vi "RGA queue listener (SubVI).vi"(0 "stop bool":refnum<vi>, 1 "binding key":string, 5 "is_running bool":refnum<vi>, 7 "log queue in":refnum<queue>, 9 "queue in":refnum<queue>, 11 "error in (no error)":errorcluster) -> (8 "error out":errorcluster)   [LabVIEW 2016]
uses:
  C:/Program Files (x86)/National Instruments/LabVIEW 2016/vi.lib/Distrio/LabbitMQ/RabbitMQ.Client.dll
  Program Files (x86)/National Instruments/LabVIEW 2016/vi.lib/Distrio/LabbitMQ/RabbitMQ.Client.dll
  global/Config_Infos.vi
  <vilib>/Distrio/LabbitMQ/Queue/Queue.lvclass
panel:
  out "after substring":string
  out "match substring":string
  out "before substring":string
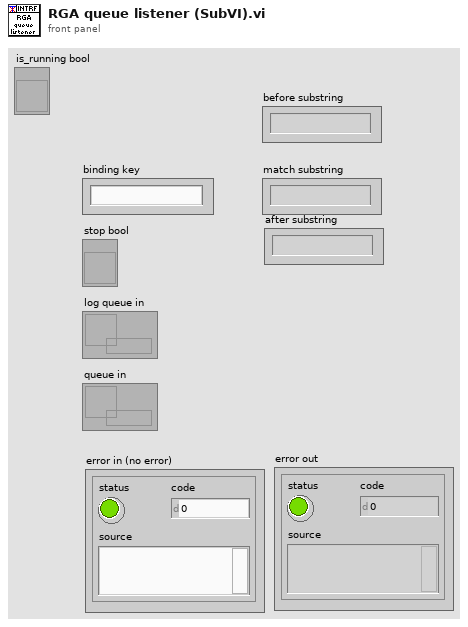
[diagram p1: front panel]
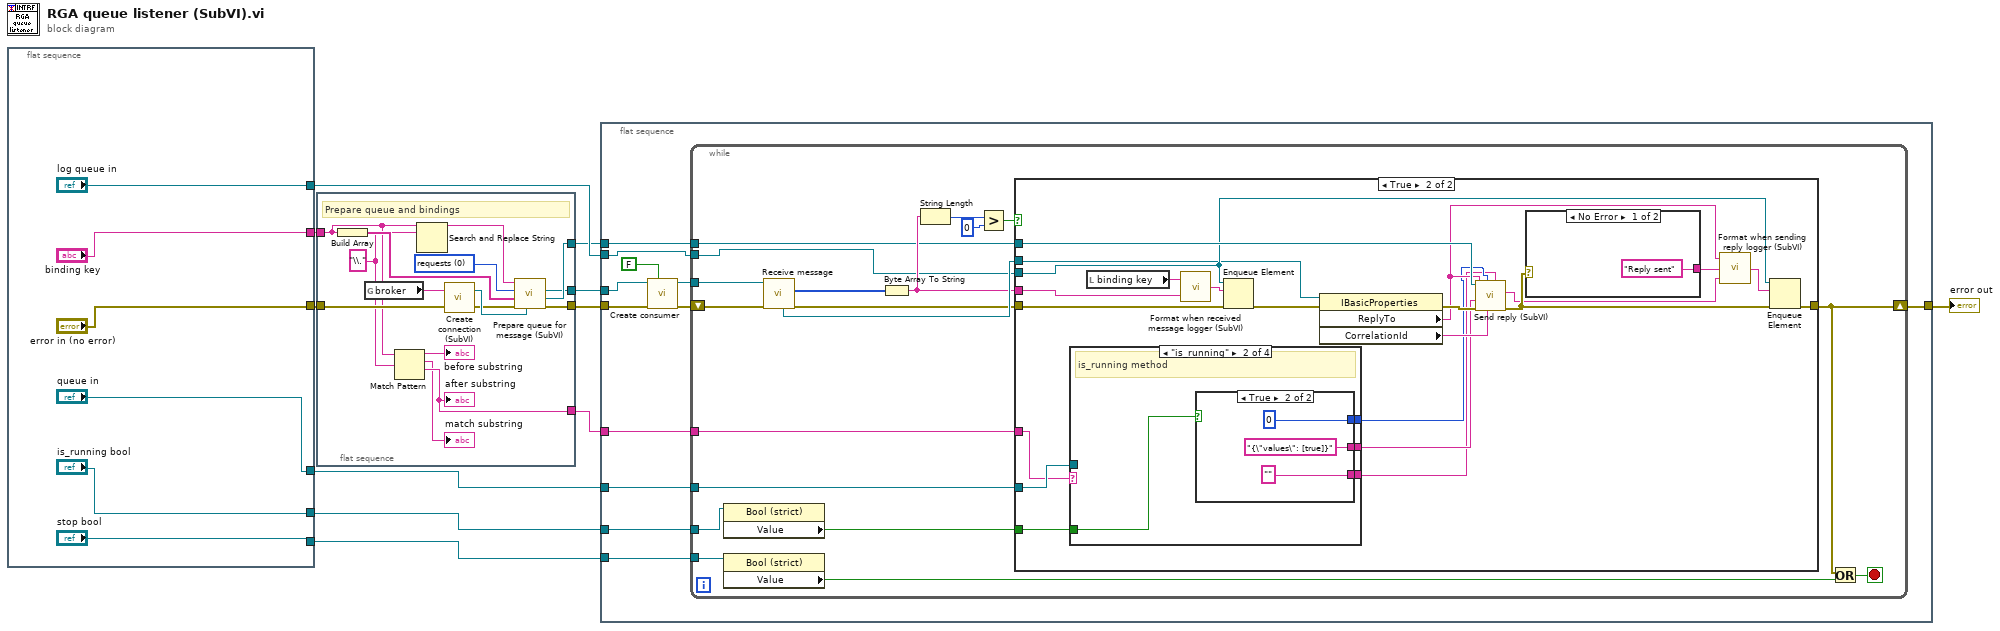
[diagram p0: block diagram]
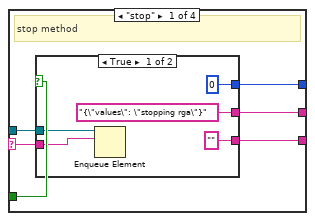
[diagram p3: hidden frame]
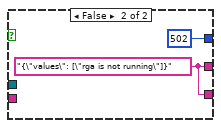
[diagram p4: hidden frame]
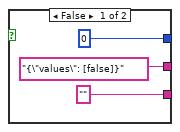
[diagram p5: hidden frame]
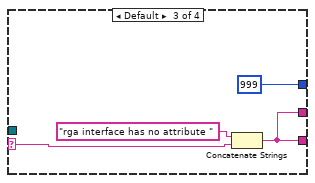
[diagram p6: hidden frame]
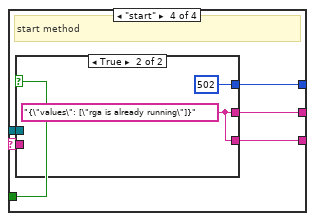
[diagram p7: hidden frame]
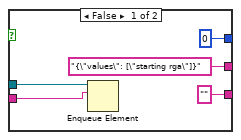
[diagram p8: hidden frame]
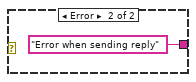
[diagram p9: hidden frame]
diagram:
  n1 = flat-sequence {
    tunnel: ["log queue in"] -> w11
    tunnel: ["queue in"] -> w10
    tunnel: ["error in (no error)"] -> w6
    tunnel: ["stop bool"] -> w5
    tunnel: ["binding key"] -> w4
    tunnel: ["is_running bool"] -> w2
    frame #0 {
    }
  }
  n2 = flat-sequence {
    tunnel: [w31] -> w9
    tunnel: [w30] -> w8
    tunnel: [w29] -> w7
    tunnel: w6 -> [w25]
    tunnel: w4 -> [w22]
    tunnel: [w21] -> w1
    frame #0 {
      w23 = "\\." ("search string")
      w26 = u16 0 items=["requests", "alerts"] ("exchange name")
      # "Prepare queue and bindings"
      n3 = Build Array(w22) -> (w32:string[])
      n4 = global read "Config_Infos.vi" "broker"() -> (w20:string)
      n5 = Match Pattern(string=w22, regular expression=w23) -> (before substring=→"before substring":string, match substring=→"match substring":string, after substring=w21:string)  [unwired: 1 in, 1 out]
      "after substring" <- w21
      n6 = Search and Replace String(input string=w22, search string=w23) -> (result string=w24:string)  [unwired: 6 in, 3 out]
      n7 = call "Create connection (SubVI).vi"("error in (no error)"=w25, "host name"=w20) -> ("error out"=w27:errorcluster, "Connection out"=w28:refnum<class "Connection.lvclass">)
      n8 = call "Prepare queue for message (SubVI).vi"("Connection in"=w28, "error in (no error)"=w27, "binding key"=w32, "exchange name"=w26, "queue \nname"=w24) -> ("error out"=w30:errorcluster, "Exchange.lvclass"=w31:refnum<class "Exchange.lvclass">, "Queue out"=w29:refnum<class "Queue.lvclass">)  [unwired: 2 out]
    }
  }
  n9 = flat-sequence {
    tunnel: w11 -> [w44]
    tunnel: w10 -> [w43]
    tunnel: w9 -> [w42]
    tunnel: w8 -> [w41]
    tunnel: w7 -> [w40]
    tunnel: w5 -> [w36]
    tunnel: [w35] -> w3
    tunnel: w2 -> [w34]
    tunnel: w1 -> [w33]
    frame #0 {
      n10 = call <vilib>:"Create consumer.vi"("noAck? (T)"=FALSE, "error in (no error)"=w41, "Queue in"=w40) -> ("error out"=w38:errorcluster, "Queue out"=w37:refnum<class "Queue.lvclass">)  [unwired: 7 in]
      n11 = while {
        tunnel: w37 -> [w63]
        shift-right: [w52] -> w35
        shift-left: w38 -> [w62]
        tunnel: w42 -> [w53]
        tunnel: w43 -> [w50]
        tunnel: w44 -> [w49]
        tunnel: w36 -> [w48]
        tunnel: w34 -> [w47]
        tunnel: w33 -> [w45]
        stop <- w54 stop-if-true
        n12 = property class="Bool (strict)"(reference=w47) -> ("Value"=w46:bool)  [unwired: 1 in, 2 out]
        n13 = property class="Bool (strict)"(reference=w48) -> ("Value"=w51:bool)  [unwired: 1 in, 2 out]
        n14 = call <vilib>:"Receive message.vi"("error in (no error)"=w62, "Consumer in"=w63) -> ("error out"=w59:errorcluster, "message body"=w61:u8[], "MessageProperties"=w60:refnum<k24>)  [unwired: 4 in, 3 out]
        n15 = Byte Array To String(unsigned byte array=w61) -> (string=w55:string)
        n16 = String Length(string=w55) -> (length=w58:i32)
        n17 = Greater?(x=w58, y=0) -> (0:w56:bool)
        n18 = case shown="True" w56 {
          tunnel: w60 -> [_ w77]
          tunnel: w55 -> [_ w86]
          tunnel: w59 -> [w64 w74]
          tunnel: [w64 w79] -> w52
          tunnel: w53 -> [_ w85]
          tunnel: w50 -> [_ w84]
          tunnel: w49 -> [_ w81]
          tunnel: w46 -> [_ w68]
          tunnel: w45 -> [_ w67]
          frame False {
          }
          frame True {
            n19 = case shown="\"is_running\"" w67 {
              selector: w67 -> [w92 _ w111 w116]
              tunnel: w84 -> [w91 _ _ w119]
              tunnel: [w89 w102 w110 w118] -> w69
              tunnel: w68 -> [w90 w103 _ w117]
              tunnel: [w88 w101 999 w115] -> w66
              tunnel: [w87 w100 w110 w114] -> w65
              frame "stop" {
                # "stop method"
                n20 = case shown="True" w90 {
                  tunnel: w91 -> [w97 _]
                  tunnel: ["{\"values\": \"stopping rga\"}" ("reply content if running") w99] -> w89
                  tunnel: w92 -> [w95 _]
                  tunnel: [0 502] -> w88
                  tunnel: ["" ("reply content if running") w99] -> w87
                  frame True {
                    n21 = Enqueue Element(queue=w97, element=w95) -> ()  [unwired: 2 in, 3 out]
                  }
                  frame False {
                    w99 = "{\"values\": [\"rga is not running\"]}" ("reply content if running")
                  }
                }
              }
              frame "is_running" {
                # "is_running method"
                n22 = case shown="True" w103 {
                  tunnel: ["{\"values\": [false]}" "{\"values\": [true]}"] -> w102
                  tunnel: [0 0] -> w101
                  tunnel: ["" ""] -> w100
                  frame False {
                  }
                  frame True {
                  }
                }
              }
              frame Default {
                n23 = Concatenate Strings("rga interface has no attribute " ("reply content if running"), w111) -> (w110:string)
              }
              frame "start" {
                # "start method"
                n24 = case shown="False" w117 {
                  tunnel: w119 -> [w124 _]
                  tunnel: ["{\"values\": [\"starting rga\"]}" ("reply content if running") w126] -> w118
                  tunnel: w116 -> [w122 _]
                  tunnel: [0 502] -> w115
                  tunnel: ["" ("reply content if running") w126] -> w114
                  frame False {
                    n25 = Enqueue Element(queue=w124, element=w122) -> ()  [unwired: 2 in, 3 out]
                  }
                  frame True {
                    w126 = "{\"values\": [\"rga is already running\"]}" ("reply content if running")
                  }
                }
              }
            }
            n26 = local read "binding key"() -> (w76:string)
            n27 = call "Format when received message logger (SubVI).vi"("received message"=w86, "queue name"=w76) -> ("info to log"=w83:string)
            n28 = Enqueue Element(queue=w81, element=w83, error in (no error)=w74) -> (error out=w73:errorcluster)  [unwired: 1 in, 2 out]
            n29 = property class="IBasicProperties"(reference=w77, error in=w73) -> (error out=w75:errorcluster, "ReplyTo"=w72:string, "CorrelationId"=w71:string)  [unwired: 1 out]
            n30 = call "Send reply (SubVI).vi"("return_msg"=w65, "Correlation ID"=w71, "retcode"=w66, "error in (no error)"=w75, "reply content"=w69, "target"=w72, "Exchange.lvclass"=w85) -> ("error out"=w80:errorcluster, "sent message"=w70:string)  [unwired: 3 in]
            n31 = case shown="No Error" w80 {
              tunnel: ["Reply sent" ("string") "Error when sending reply" ("string")] -> w82
              frame No Error {
              }
              frame Error {
              }
            }
            n32 = call "Format when sending reply logger (SubVI).vi"("sent message"=w70, "status"=w82, "queue name"=w72) -> ("info to log"=w78:string)
            n33 = Enqueue Element(queue=w81, element=w78, error in (no error)=w80) -> (error out=w79:errorcluster)  [unwired: 1 in, 2 out]
          }
        }
        n34 = Or(x=w52, y=w51) -> (x .or. y?=w54:bool)
      }
    }
  }
  "error out" <- w3
